vi "RegExJitSubstitude.vi"(4 "MatchOptions":u32 format="%.0x", 5 "JitCompileOptions":u32 format="%.0x", 6 "Offset":i32, 7 "CompileOptions":u32 format="%.0x", 8 "error in":errorcluster, 9 "Replacement":string, 10 "search pattern":string, 11 "Subject":string) -> (0 "error out":errorcluster, 3 "OutString":string)   [LabVIEW 2021, in "libpcre2-8.lvlib"]
uses:
  libpcre2-8.lvlib
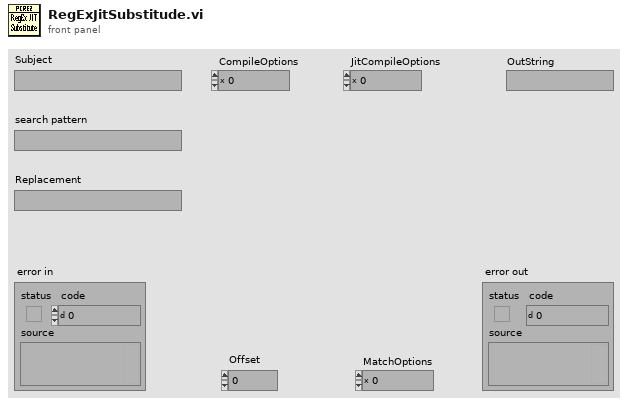
[diagram p1: front panel]
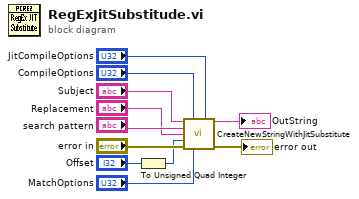
[diagram p0: block diagram]
diagram:
  n1 = To Unsigned Quad Integer(1:"Offset") -> (0:w1:u64)
  n2 = call "CreateNewStringWithJitSubstitute.vi"("Subject"="Subject", "CompileOptions"="CompileOptions", "JitCompileOptions"="JitCompileOptions", "search pattern"="search pattern", "Replacement"="Replacement", "Offset"=w1, "error in"="error in", "MatchOptions"="MatchOptions") -> ("OutString"=→"OutString":string, "error out"=→"error out":errorcluster)  [unwired: 6 in]
